vi "place_runner_in_maze_start.vi"(0 "maze with runner in":T3[][](array[typedef]), 11 "state":T1={"State"=enum."sense", "Maze"=[[FALSE, FALSE, FALSE, FALSE, FALSE, FALSE, FALSE, FALSE, FALSE], [FALSE, FALSE, TRUE, FALSE, FALSE, TRUE, TRUE, TRUE, FALSE], [FALSE, FALSE, TRUE, TRUE, TRUE, TRUE, FALSE, FALSE, FALSE], [FALSE, FALSE, TRUE, FALSE, FALSE, TRUE, FALSE, FALSE, FALSE], [TRUE, TRUE, TRUE, FALSE, FALSE, TRUE, FALSE, TRUE, TRUE], [FALSE, FALSE, FALSE, TRUE, TRUE, TRUE, FALSE, TRUE, FALSE], [FALSE, FALSE, FALSE, FALSE, FALSE, TRUE, TRUE, TRUE, FALSE], [FALSE, FALSE, FALSE, FALSE, FALSE, FALSE, FALSE, FALSE, FALSE], [FALSE, FALSE, FALSE, FALSE, FALSE, FALSE, FALSE, FALSE, FALSE]], "Runner Row"=0, "Runner Column"=1, "Runner Direction"=enum."east", "Sense"={"wall in front"=FALSE, "wall to left"=FALSE, "wall to right"=FALSE, "wall behind"=FALSE, "exit column"=FALSE}, "Hand"=enum."Left-handed"}) -> (4 "maze with runner out":T3[][](array[typedef]))   [LabVIEW 2016]
doc: "Updates the direction of the mouse then places the cheese in the last open row of last column in the maze.\n\nMuhannad Alghamdi\nCSUSB Physics 350"
uses:
  typedefs/cell_typedef.ctl
  typedefs/state.ctl
  typedefs/action_start.ctl
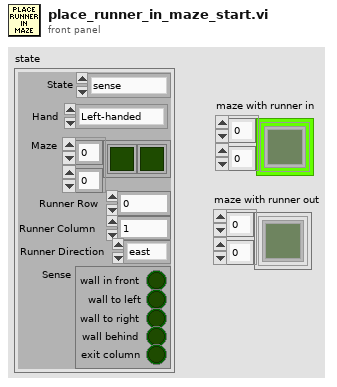
[diagram p1: front panel]
types:
  T1 = typedef "state.ctl" = cluster{"State":T2, "Maze":bool[][], "Runner Row":i32, "Runner Column":i32, "Runner Direction":enum16{"east", "north", "west", "south"}, "Sense":cluster{"wall in front":bool, "wall to left":bool, "wall to right":bool, "wall behind":bool, "exit column":bool}, "Hand":enum16{"Left-handed", "Right-handed"}}
  T2 = typedef "action_start.ctl" = enum16{"sense", "decide", "step", "pivot right", "pivot left", "stop"}
  T3 = typedef "cell_typedef.ctl" = cluster{"open":bool, "runner":u16}
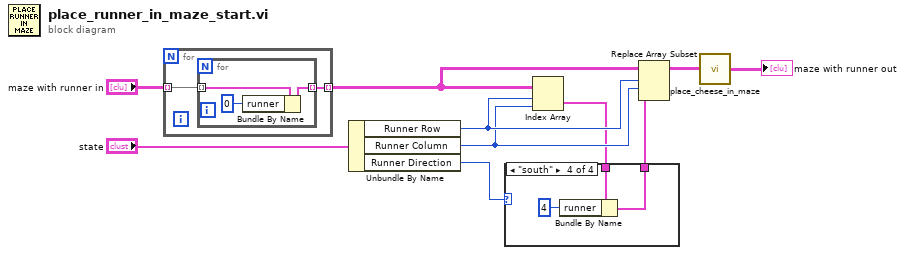
[diagram p0: block diagram]
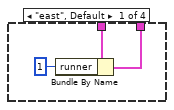
[diagram p2: hidden frame]
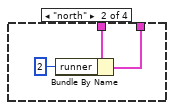
[diagram p3: hidden frame]
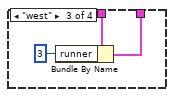
[diagram p4: hidden frame]
diagram:
  n1 = for {
    tunnel: "maze with runner in" -> [w12] mode=indexing
    tunnel: [w11] -> w9 mode=indexing
    n2 = for {
      tunnel: w12 -> [w15] mode=indexing
      tunnel: [w14] -> w11 mode=indexing
      n3 = Bundle By Name(cluster=w15, "runner"=u16 0) -> (w14:T3)
    }
  }
  n4 = Unbundle By Name("state") -> ("Runner Row"=w7:i32, "Runner Column"=w6:i32, "Runner Direction"=w5:enum16{"east", "north", "west", "south"})
  n5 = Index Array(array=w9, index (row)=w7, index (col)=w6) -> (element=w4:T3)
  n6 = case shown="\"south\"" w5 {
    tunnel: w4 -> [w17 w20 w23 w26]
    tunnel: [w16 w19 w22 w25] -> w3
    frame "east", Default {
      n7 = Bundle By Name(cluster=w17, "runner"=u16 1) -> (w16:T3)
    }
    frame "north" {
      n8 = Bundle By Name(cluster=w20, "runner"=u16 2) -> (w19:T3)
    }
    frame "west" {
      n9 = Bundle By Name(cluster=w23, "runner"=u16 3) -> (w22:T3)
    }
    frame "south" {
      n10 = Bundle By Name(cluster=w26, "runner"=u16 4) -> (w25:T3)
    }
  }
  n11 = Replace Array Subset(array=w9, new element=w3, index (row)=w7, index (col)=w6) -> (w1:T3[][])
  n12 = call "place_cheese_in_maze.vi"("Array in"=w1) -> ("Array out"=→"maze with runner out":T3[][])
